vi "Status.vi"(8 "error in":errorcluster, 11 "VISA resource name in":refnum<visa-resource-name>) -> (0 "error out":errorcluster, 2 "Status":string, 3 "VISA resource name out":refnum<visa-resource-name>)   [LabVIEW 2021, in "Keysight U1282A.lvlib"]
doc: "El comando de estatus del instrumento (STAT?) regresa el estatus del instrumento U1281A/U1282A como un cluster de datos."
uses:
  Keysight U1282A.lvlib
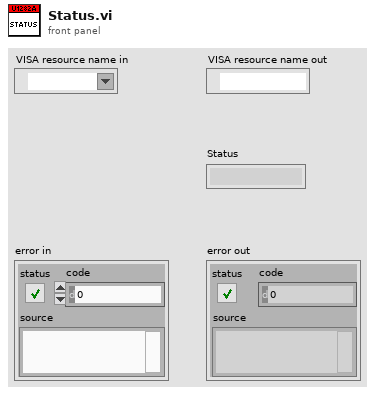
[diagram p1: front panel]
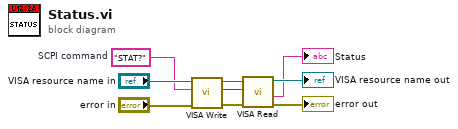
[diagram p0: block diagram]
diagram:
  w3 = "STAT?"  # SCPI command
  n1 = call "VISA Write.vi"("error in"="error in", "SCPI command"=w3, "VISA resource in"="VISA resource name in") -> ("error out"=w9:errorcluster, "Bytes at Port out"=w8:u32, "VISA resource out"=w7:refnum<visa-resource-name>)  [unwired: 6 in]
  n2 = call "VISA Read.vi"("error in"=w9, "Bytes at Port in"=w8, "VISA resource in"=w7) -> ("error out"=→"error out":errorcluster, "Reading"=→"Status":string, "VISA resource out"=→"VISA resource name out":refnum<visa-resource-name>)  [unwired: 5 in, 1 out]
